vi "Un-suspend heater.vi"(6 "D":dbl, 8 "error in (no error)":errorcluster, 9 "I":dbl, 10 "P":dbl, 11 "VISA Refnum in":refnum<visa-resource-name>) -> (0 "error out":errorcluster, 3 "VISA Refnum out":refnum<visa-resource-name>)   [LabVIEW 2015]
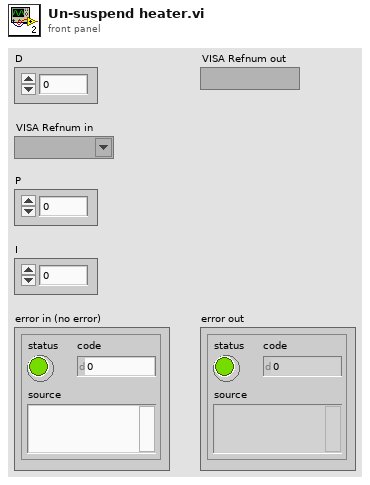
[diagram p1: front panel]
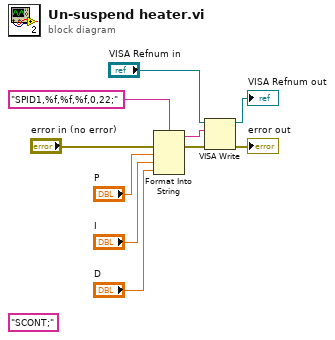
[diagram p0: block diagram]
diagram:
  (unwired) "SCONT;" ("write buffer")
  n1 = Format Into String(format string="SPID1,%f,%f,%f,0,22;", error in="error in (no error)", "P", "I", "D") -> (resulting string=w8:string, error out=w7:errorcluster)  [unwired: 1 in]
  n2 = VISA Write(VISA resource name="VISA Refnum in", write buffer=w8, error in (no error)=w7) -> (VISA resource name out=→"VISA Refnum out":refnum<visa-resource-name>, error out=→"error out":errorcluster)  [unwired: 1 out]
